vi "5.6.vi"() -> ()   [LabVIEW 2017]
uses:
  <vilib>/measure/NI_MABase.lvlib
panel:
  out "y大小":i32
  out "y最大值":dbl
  out "dt":dbl
  out "波形图":waveform(dbl)(graph)
  in  "sampling info":cluster{"Fs":dbl, "#s":dbl}={"Fs"=1000.0, "#s"=1000.0} caption="采样信息" {"Fs" format="%.2p"}
  in  "phase":dbl caption="相位" format="%.2p"
  in  "frequency":dbl=10.0 caption="频率" format="%0.2p"
  in  "amplitude":dbl=1.0 caption="幅值" format="%0.2p"
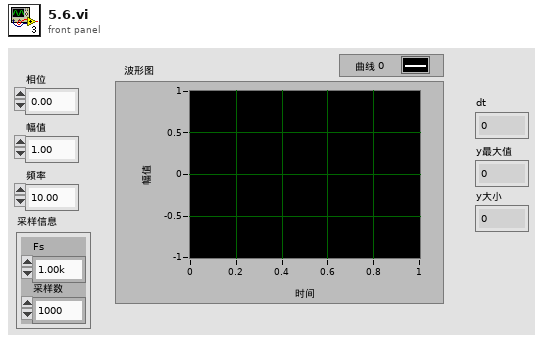
[diagram p1: front panel]
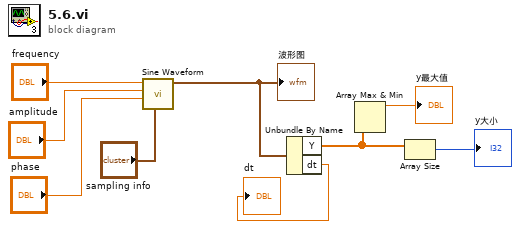
[diagram p0: block diagram]
diagram:
  n1 = call <vilib>:"Sine Waveform.vi"("sampling info"="sampling info", "phase"="phase", "amplitude"="amplitude", "frequency"="frequency") -> ("signal out"=w5:waveform(dbl))  [unwired: 6 in, 1 out]
  "波形图" <- w5
  n2 = Unbundle By Name(w5) -> ("Y"=w2:dbl[], "dt"=→"dt":dbl)
  n3 = Array Max & Min(array=w2) -> (max value=→"y最大值":dbl)  [unwired: 3 out]
  n4 = Array Size(array=w2) -> (size(s)=→"y大小":i32)
